vi "Decompose Poll Source Code Cron String.vi"(11 "String":string) -> (3 "Source Code Poll":T1)   [LabVIEW 2014]
uses:
  Controls/Source Code Control Selection - STYP.ctl
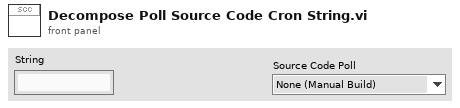
[diagram p1: front panel]
types:
  T1 = typedef "Source Code Control Selection - STYP.ctl" = enum16{"None (Manual Build)", "Every 15 Minutes", "Every 30 Minutes", "Every 45 Minutes", "Every Hour", "Every 2 Hours", "Everyday "}
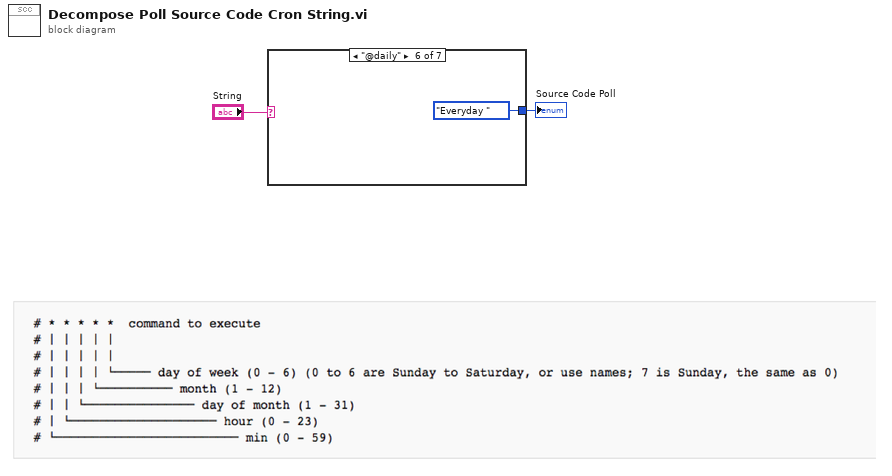
[diagram p0: block diagram]
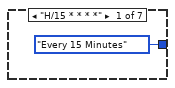
[diagram p2: hidden frame]
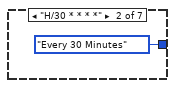
[diagram p3: hidden frame]
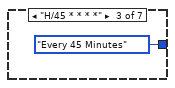
[diagram p4: hidden frame]
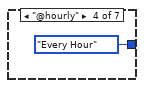
[diagram p5: hidden frame]
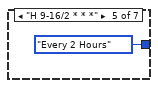
[diagram p6: hidden frame]
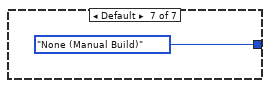
[diagram p7: hidden frame]
diagram:
  n1 = case shown="\"@daily\"" "String" {
    tunnel: [Source_Code_Control_Selection_-_STYP."Every 15 Minutes" ("Source Code Poll") Source_Code_Control_Selection_-_STYP."Every 30 Minutes" ("Source Code Poll") Source_Code_Control_Selection_-_STYP."Every 45 Minutes" ("Source Code Poll") Source_Code_Control_Selection_-_STYP."Every Hour" ("Source Code Poll") Source_Code_Control_Selection_-_STYP."Every 2 Hours" ("Source Code Poll") Source_Code_Control_Selection_-_STYP."Everyday " ("Source Code Poll") Source_Code_Control_Selection_-_STYP."None (Manual Build)" ("Source Code Poll")] -> w1
    frame "H/15 * * * *" {
    }
    frame "H/30 * * * *" {
    }
    frame "H/45 * * * *" {
    }
    frame "@hourly" {
    }
    frame "H 9-16/2 * * *" {
    }
    frame "@daily" {
    }
    frame Default {
    }
  }
  "Source Code Poll" <- w1
